vi "data_sonar.vi"() -> ()   [LabVIEW 2021]
panel:
  in  "dt":u32
  in  "stop":bool
  out "Waveform Graph":dbl[](graph)
  in  "scale":dbl
  out "Numeric 2":i32
  in  "Numeric":i32
  out "Intensity Graph":dbl[][](graph)
  in  "data 2":T1={"Waveform(s)"=[{"relativeInitialX"=-1.5939337890625172e-05, "xIncrement"=1e-07, "wfm"=array[1000 elements]}], "Actual Record Length"=1000, "Actual Sample Rate"=10000000.0, "Auto Triggered"=FALSE} {"Actual Sample Rate" format="%#.2p"}
  # "17.3u > 50mm = 0.346 / 2.87 \n7.46u   > 30mm = 0.24 /"
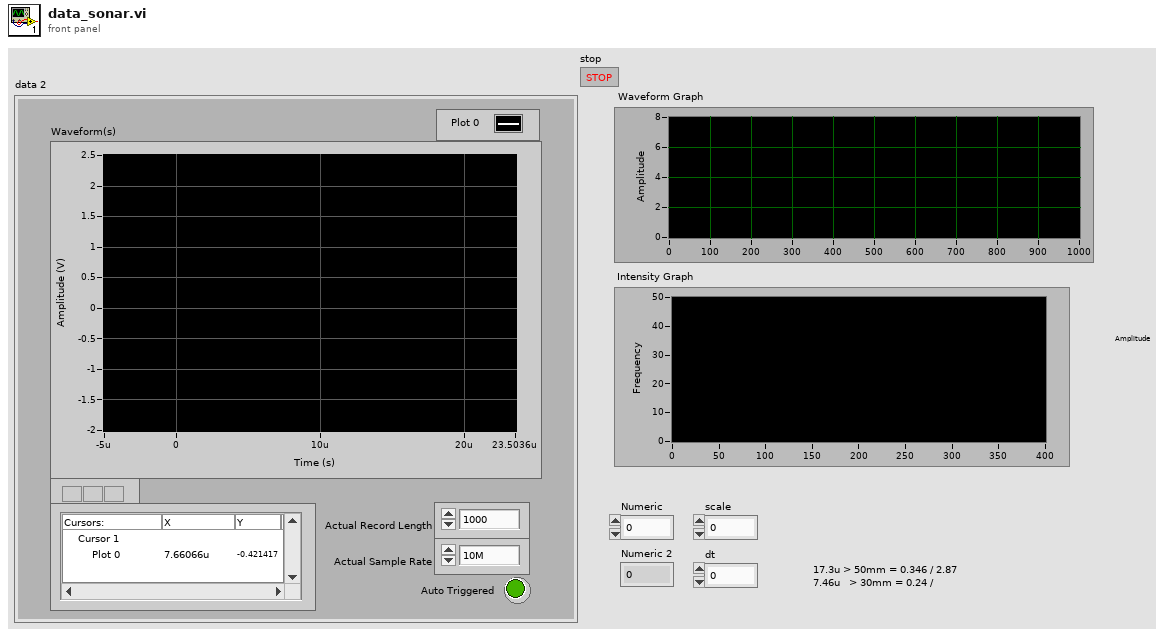
[diagram p1: front panel]
types:
  T1 = cluster{"Waveform(s)":cluster{"relativeInitialX":dbl, "xIncrement":dbl, "wfm":dbl[]}[], "Actual Record Length":i32, "Actual Sample Rate":dbl, "Auto Triggered":bool}
  T2 = cluster{"relativeInitialX":dbl, "xIncrement":dbl, "wfm":dbl[]}[]
  T3 = cluster{"relativeInitialX":dbl, "xIncrement":dbl, "wfm":dbl[]}
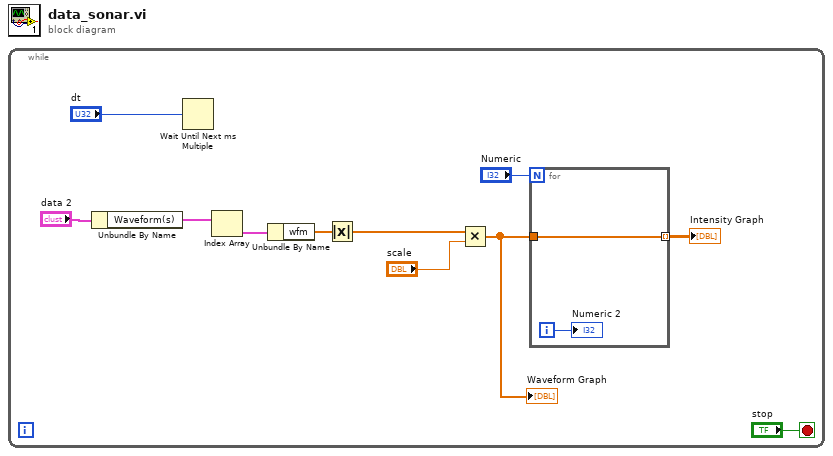
[diagram p0: block diagram]
diagram:
  n1 = while {
    stop <- "stop" stop-if-true
    n2 = Unbundle By Name("data 2") -> ("Waveform(s)"=w10:T2)
    n3 = Wait Until Next ms Multiple(millisecond multiple="dt") -> ()  [unwired: 1 out]
    n4 = Index Array(array=w10) -> (element=w9:T3)  [unwired: 1 in]
    n5 = Unbundle By Name(w9) -> ("wfm"=w6:dbl[])
    n6 = Absolute Value(x=w6) -> (abs(x)=w4:dbl[])
    n7 = Multiply(x=w4, y="scale") -> (x*y=w3:dbl[])
    "Waveform Graph" <- w3
    n8 = for {
      N: "Numeric" -> [_]
      tunnel: w3 -> [w13]
      tunnel: [w13] -> w7 mode=indexing
      i -> [w12]
      "Numeric 2" <- w12
    }
    "Intensity Graph" <- w7
  }
